vi "remove dead functions.vi"(9 "command in":string[](array[string]), 10 "old sensor datas":T1, 11 "sensor datas":T1) -> (3 "remove":bool)   [LabVIEW 2011]
panel:
  out "accessed value 2":dbl
  out "accessed value":dbl
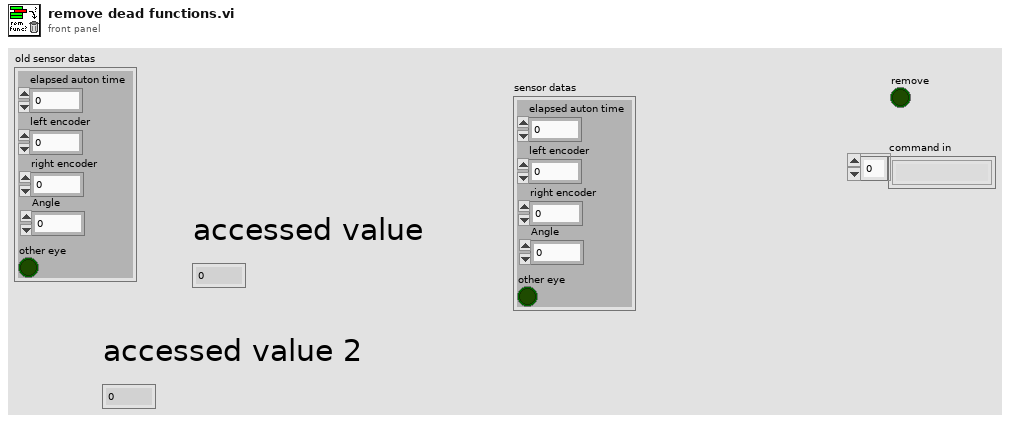
[diagram p1: front panel]
types:
  T1 = cluster{"elapsed auton time":dbl, "left encoder":dbl, "other eye":bool, "right encoder":dbl, "Angle":dbl}
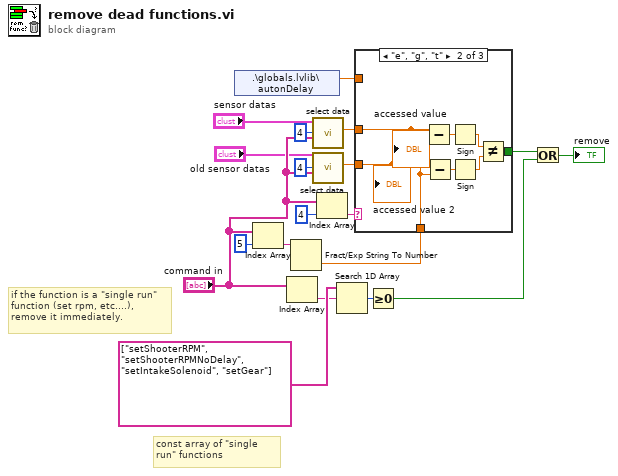
[diagram p0: block diagram]
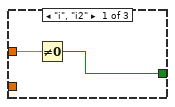
[diagram p2: hidden frame]
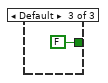
[diagram p3: hidden frame]
diagram:
  # "const array of \"single run\" functions"
  # "if the function is a \"single run\" function (set rpm, etc....), remove it immediately."
  n1 = shared-variable ".\\globals.lvlib\\autonDelay"() -> (w3:dbl)  [unwired: 1 in, 1 out]
  n2 = Index Array(array="command in", index=5) -> (element=w10:string)
  n3 = Index Array(array="command in") -> (element=w18:string)  [unwired: 1 in]
  n4 = Fract/Exp String To Number(string=w10) -> (number=w9:dbl)  [unwired: 3 in, 1 out]
  n5 = call "select data.vi"("command and parameters in"="command in", "index"=u8 4, "sensor datas"="sensor datas") -> ("accessed value"=w7:dbl)  [unwired: 8 in]
  n6 = call "select data.vi"("command and parameters in"="command in", "index"=u8 4, "sensor datas"="old sensor datas") -> ("accessed value"=w12:dbl)  [unwired: 8 in]
  n7 = Index Array(array="command in", index=4) -> (element=w6:string)
  n8 = Search 1D Array(1D array=string[] ["setShooterRPM", "setShooterRPMNoDelay", "setIntakeSolenoid", "setGear"], element=w18) -> (index of element=w17:i32)  [unwired: 1 in]
  n9 = case shown="\"e\", \"g\", \"t\"" w6 {
    tunnel: w12 -> [_ w22 _]
    tunnel: w9 -> [_ w25 _]
    tunnel: [w20 w24 FALSE] -> w8
    tunnel: w7 -> [w21 w23 _]
    tunnel: w3 -> [_ _ _]
    frame "i", "i2" {
      n10 = Not Equal To 0?(x=w21) -> (x != 0?=w20:bool)
    }
    frame "e", "g", "t" {
      n11 = Subtract(x=w23, y=w25) -> (x-y=w29:dbl)
      n12 = Subtract(x=w22, y=w25) -> (x-y=w28:dbl)
      n13 = Sign(1:w29) -> (0:w27:dbl)
      n14 = Sign(1:w28) -> (0:w26:dbl)
      n15 = Not Equal?(x=w27, y=w26) -> (x != y?=w24:bool)
      "accessed value" <- w23
      "accessed value 2" <- w22
    }
    frame Default {
    }
  }
  n16 = Greater Or Equal To 0?(x=w17) -> (x >= 0?=w16:bool)
  n17 = Or(x=w8, y=w16) -> (x .or. y?=→"remove":bool)
